vi "显示测试结果-拧紧程式序号.vi"(9 "拧紧程式序号数组":i32[](array[numeric]), 11 "Img输入":T1) -> ()   [LabVIEW 2014]
uses:
  <vilib>/vision/Image Controls.llb/IMAQ Image.ctl
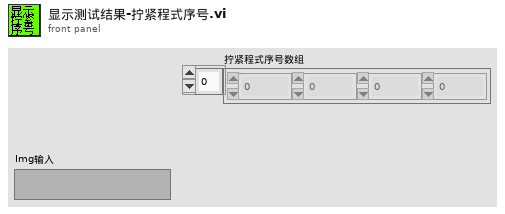
[diagram p1: front panel]
types:
  T1 = typedef "IMAQ Image.ctl" = refnum<image>
  T2 = cluster{"Desired Font (Application)":enum16{"User-specified Font", "Application Font", "System Font", "Dialog Font"}, "[User-specified Font]":cluster{"Font Name":string, "Size":i16, "Strikeout?":bool, "Italic?":bool, "Underline?":bool, "Outline?":bool, "Shadow?":bool, "Bold?":bool, "Rotation Angle":dbl}, "Horizontal Alignment":i16, "Vertical Alignment":i16}
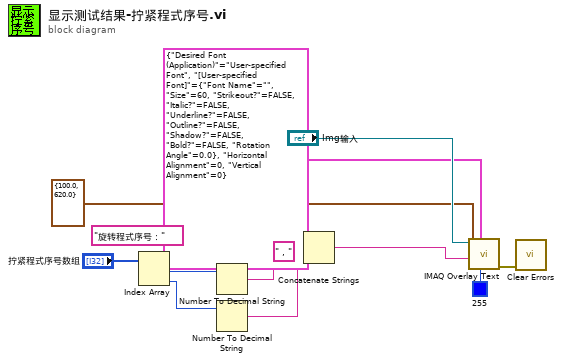
[diagram p0: block diagram]
diagram:
  n1 = Index Array(array="拧紧程式序号数组") -> (element #1=w3:i32, element #2=w2:i32)  [unwired: 2 in]
  n2 = Number To Decimal String(number=w3) -> (decimal integer string=w6:string)  [unwired: 1 in]
  n3 = Number To Decimal String(number=w2) -> (decimal integer string=w1:string)  [unwired: 1 in]
  n4 = Concatenate Strings("旋转程式序号：", w6, " , " ("字符串"), w1) -> (w9:string)
  n5 = call "IMAQ Overlay Text"("Text Color (black)"=u32 255, "Font, Size & Style"=T2 {"Desired Font (Application)"=enum."User-specified Font", "[User-specified Font]"={"Font Name"="", "Size"=60, "Strikeout?"=FALSE, "Italic?"=FALSE, "Underline?"=FALSE, "Outline?"=FALSE, "Shadow?"=FALSE, "Bold?"=FALSE, "Rotation Angle"=0.0}, "Horizontal Alignment"=0, "Vertical Alignment"=0}, "String"=w9, "Origin"=cluster{dbl, "Numeric":dbl} {100.0, "Numeric"=620.0}, "Image"="Img输入") -> ("error out"=w10:errorcluster)  [unwired: 5 in, 1 out]
  n6 = call <vilib>:"Clear Errors.vi"("error in (no error)"=w10) -> ()  [unwired: 5 in, 2 out]
